vi "Retrieve SubComponent Data.vi"(5 "Component ID":u8, 7 "FPGA Interface":refnum<class "FPGA Interface.lvclass">, 8 "error in (no error)":errorcluster, 11 "1553 SubComponent in":refnum<class "1553 SubComponent.lvclass">) -> (0 "error out":errorcluster, 3 "1553 SubComponent out":refnum<class "1553 SubComponent.lvclass">)   [LabVIEW 2020, in "BCI-1553 API.lvlib" / "1553 SubComponent.lvclass"]
doc: "Retrieves all the parameters from the 1553 Session component. A read must be called after this to retrieve the specific parameter values."
uses:
  1553 SubComponent.lvclass
  Dependencies/FPGA Interface/FPGA Interface.lvclass
  1553 SubComponent.lvclass/1553 SubComponent.ctl
  Dependencies/Registry/Registry.lvclass/Registry.ctl
  Frames & Messages/TypeDefs/Parameter Table Data.ctl
  Frames & Messages/TypeDefs/Scaling Information.ctl
  Dependencies/Registry/Add Entry.vi
  Dependencies/Registry/Registry.lvclass
  BCI-1553 API.lvlib
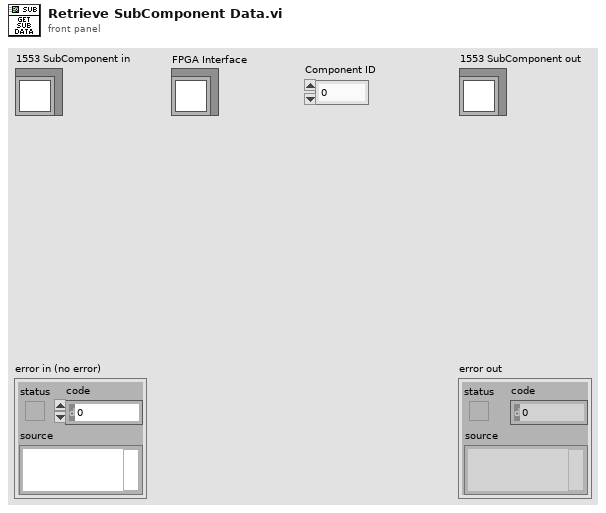
[diagram p1: front panel]
types:
  T1 = typedef "BCI-1553 API.lvlib/Parameter Table Data.ctl" = cluster{"Parameter Name":string, "Base Word":u16, "Address":u16, "Value":u64, "Mask":u16[], "Scaling Info":T2}
  T2 = typedef "BCI-1553 API.lvlib/Scaling Information.ctl" = cluster{"Bit Offset":i32, "Bit Count":i32, "LSB Resolution":dbl, "2's Complement":bool, "Big Endian":bool, "Sign Bit":bool}
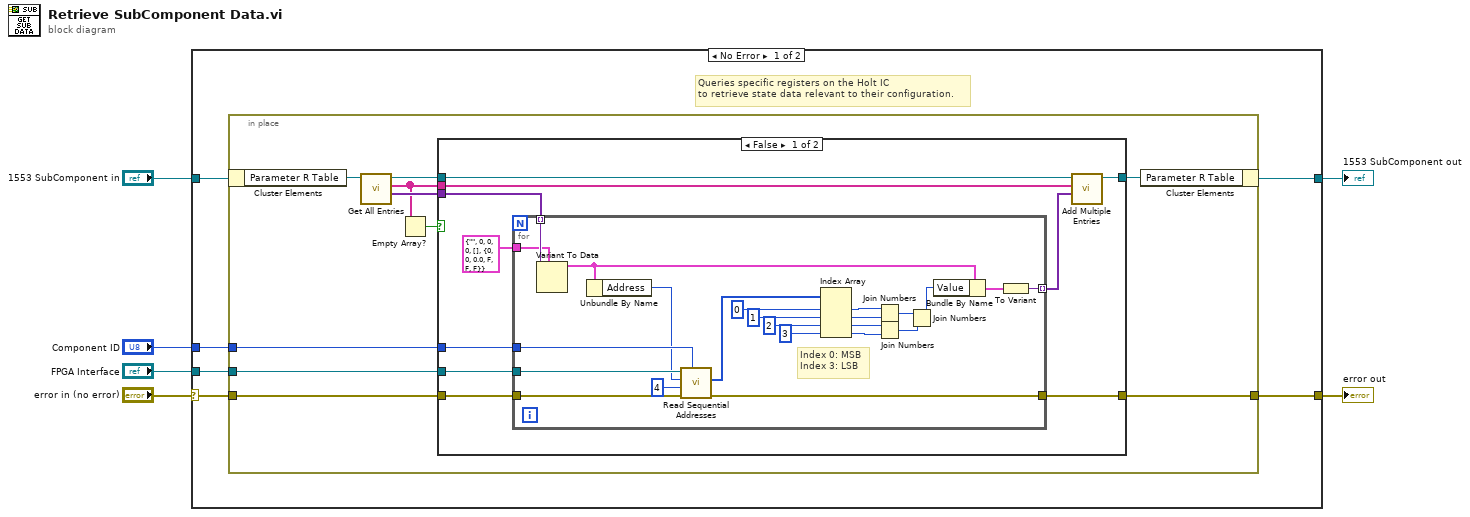
[diagram p0: block diagram]
diagram:
  n1 = case shown="No Error" "error in (no error)" {
    selector: "error in (no error)" -> [w12 w58]
    tunnel: [w9 w58] -> w5
    tunnel: [w7 w57] -> w3
    tunnel: "1553 SubComponent in" -> [w8 w57]
    tunnel: "FPGA Interface" -> [w11 _]
    tunnel: "Component ID" -> [w10 _]
    frame No Error {
      # "Queries specific registers on the Holt IC\nto retrieve state data relevant to their configuration."
      n2 = in-place {
        in-place-border: w12 -> [w20]
        in-place-border: w11 -> [w19]
        in-place-border: w10 -> [w18]
        in-place-border: [w17] -> w9
        n3 = in-place-cluster #1(w8) -> ("Parameter R Table"=w15:refnum<class "Registry.lvclass">)
        n4 = call "Get All Entries.vi"("Registry in"=w15) -> ("Values"=w21:variant[], "Keys"=w14:string[])  [unwired: 8 in, 1 out]
        n5 = Empty Array?(array=w14) -> (empty?=w13:bool)
        n6 = case shown="False" w13 {
          tunnel: w21 -> [w31 _]
          tunnel: w20 -> [w30 w55]
          tunnel: w19 -> [w29 _]
          tunnel: w18 -> [w28 _]
          tunnel: [w27 w55] -> w17
          tunnel: [w25 w56] -> w16
          tunnel: w15 -> [w24 w56]
          tunnel: w14 -> [w23 _]
          frame False {
            n7 = for {
              tunnel: w31 -> [w54] mode=indexing
              tunnel: w30 -> [w52]
              tunnel: w29 -> [w53]
              tunnel: w28 -> [w51]
              tunnel: [w49] -> w27
              tunnel: [w47] -> w26 mode=indexing
              tunnel: T1 {"Parameter Name"="", "Base Word"=0, "Address"=0, "Value"=0, "Mask"=[], "Scaling Info"={"Bit Offset"=0, "Bit Count"=0, "LSB Resolution"=0.0, "2's Complement"=FALSE, "Big Endian"=FALSE, "Sign Bit"=FALSE}} ("Parameter Table Data") -> [w32]
              # "Index 0: MSB\nIndex 3: LSB"
              n8 = Variant To Data(type=w32, Variant=w54) -> (data=w48:T1)  [unwired: 1 in, 1 out]
              n9 = Unbundle By Name(w48) -> ("Address"=w50:u16)
              n10 = call-dynamic "Read Sequential Addresses.vi"("Target IC (1-8)"=w51, "error in (no error)"=w52, "Addresses to Read"=u16 4, "Starting Address"=w50, "FPGA Interface in"=w53) -> ("error out"=w49:errorcluster, "Data"=w46:u16[])  [unwired: 5 in]
              n11 = Index Array(array=w46, index #1=0 ("index"), index #2=1 ("index"), index #3=2 ("index"), index #4=3 ("index")) -> (element #1=w38:u16, element #2=w37:u16, element #3=w36:u16, element #4=w35:u16)
              n12 = Join Numbers(hi=w38, lo=w37) -> ((hi.lo)=w45:u32)
              n13 = Join Numbers(hi=w36, lo=w35) -> ((hi.lo)=w44:u32)
              n14 = Join Numbers(hi=w45, lo=w44) -> ((hi.lo)=w43:u64)
              n15 = Bundle By Name(cluster=w48, "Value"=w43) -> (w34:T1)
              n16 = To Variant(anything=w34) -> (Variant=w47:variant)
            }
            n17 = call "Add Multiple Entries.vi"("Values"=w26, "Keys"=w23, "Registry in"=w24) -> ("Registry out"=w25:refnum<class "Registry.lvclass">)  [unwired: 6 in, 2 out]
          }
          frame True {
            # "No op if there are no parameters."
          }
        }
        n18 = in-place-cluster #1("Parameter R Table"=w16) -> (w7:refnum<class "1553 SubComponent.lvclass">)
      }
    }
    frame Error {
    }
  }
  "error out" <- w5
  "1553 SubComponent out" <- w3
